vi "SSFG_simple.vi"() -> ()   [LabVIEW 2014]
uses:
  <vilib>/Utility/error.llb/DialogType.ctl
  <vilib>/DAQmx/write.llb/DAQmx Write (Analog Wfm 1Chan NSamp).vi
  <vilib>/DAQmx/create/channels.llb/DAQmx Create Channel (AO-Voltage-Basic).vi
  <vilib>/DAQmx/configure/timing.llb/DAQmx Timing (Sample Clock).vi
  <vilib>/DAQmx/miscellaneous.llb/DAQmx Fill In Error Info.vi
  <resource>/objmgr/daqmx.rc
  <vilib>/measure/NI_MABase.lvlib
panel:
  out "Waveform Graph 2":waveform(dbl)(graph)
  in  "Power Signal Parameters":T1={"Waveform Type"=0, "Amplitude"=1.0, "Frequency"=17.0} {"Frequency" format="%0.2p"; "Waveform Type" items=["Sine Wave", "Triangle Wave", "Square Wave", "Sawtooth Wave"]}
  in  "Number of Samples/Cycle":dbl=1000.0
  in  "Stop":bool
  in  "Update Rate":dbl=1000.0 format="%0.2f"
  in  "Physical Channel":tag
  in  "Power Signal":bool
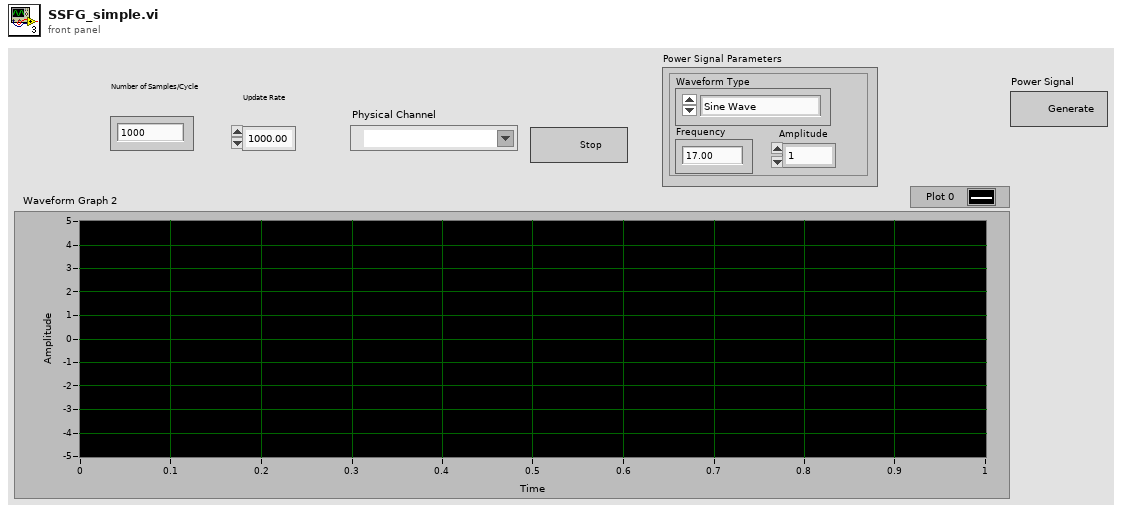
[diagram p1: front panel]
types:
  T1 = cluster{"Waveform Type":u16, "Amplitude":dbl, "Frequency":dbl}
  T2 = typedef "DialogType.ctl" = u16
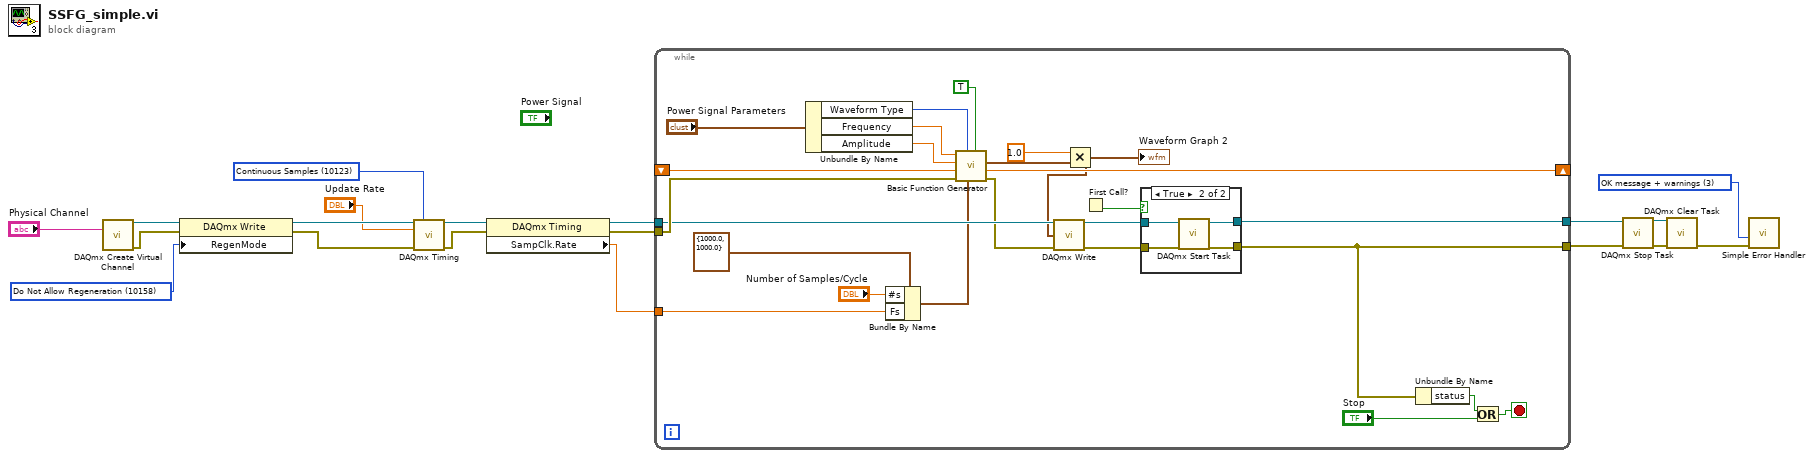
[diagram p0: block diagram]
diagram:
  w8 = T2 3 items=["no dialog", "OK message", "continue or stop message", "OK message + warnings", "continue/stop + warnings"] ("type of dialog (OK msg:1)")
  w13 = 10123 items=["Finite Samples"=10178, "Continuous Samples"=10123, "Hardware Timed Single Point"=12522] ("sample mode")
  w14 = 10158 items=["Allow Regeneration"=10097, "Do Not Allow Regeneration"=10158] ("RegenMode")
  n1 = call-poly <vilib>:"DAQmx Create Virtual Channel.vi"("physical channels"="Physical Channel") -> ("task out"=w18:refnum<k21>, "error out"=w16:errorcluster)  [unwired: 13 in]
  n2 = property class="DAQmx Write"(reference=w18, error in=w16, "RegenMode"=w14) -> (reference out=w17:refnum<k21>, error out=w15:errorcluster)
  n3 = call-poly <vilib>:"DAQmx Timing.vi"("task/channels in"=w17, "sample mode"=w13, "rate"="Update Rate", "error in"=w15) -> ("task out"=w11:refnum<k21>, "error out"=w10:errorcluster)  [unwired: 10 in]
  n4 = property class="DAQmx Timing"(reference=w11, error in=w10) -> (reference out=w2:refnum<k21>, error out=w1:errorcluster, "SampClk.Rate"=w9:dbl)
  n5 = while "while" {
    tunnel: w1 -> [w44]
    tunnel: w9 -> [w42]
    tunnel: w2 -> [w41]
    tunnel: [w36] -> w4
    tunnel: [w35] -> w3
    shift-right: [w23] -> _
    shift-left: _ -> [w22]
    stop <- w33 stop-if-true
    n6 = Unbundle By Name("Power Signal Parameters") -> ("Waveform Type"=w29:u16, "Frequency"=w28:dbl, "Amplitude"=w27:dbl)
    n7 = Bundle By Name(cluster=cluster{"Fs":dbl, "#s":dbl} {"Fs"=1000.0, "#s"=1000.0} ("sampling info"), "#s"="Number of Samples/Cycle", "Fs"=w42) -> (w30:cluster{"Fs":dbl, "#s":dbl})
    n8 = call <vilib>:"Basic Function Generator.vi"("reset signal"=TRUE, "sampling info"=w30, "signal type"=w29, "error in (no error)"=w44, "phase"=w22, "amplitude"=w27, "frequency"=w28) -> ("error out"=w38:errorcluster, "phase out"=w23:dbl, "signal out"=w25:waveform(dbl))  [unwired: 2 in]
    n9 = Multiply(x=1.0 ("y"), y=w25) -> (x*y=w20:waveform(dbl))
    "Waveform Graph 2" <- w20
    n10 = call-poly <vilib>:"DAQmx Write.vi"("task/channels in"=w41, "data"=w20, "error in"=w38) -> ("task out"=w40:refnum<k21>, "error out"=w39:errorcluster)  [unwired: 10 in, 1 out]
    n11 = First Call?() -> (First Call?: T/F=w37:bool)
    n12 = case shown="True" w37 {
      tunnel: w40 -> [w45 w50]
      tunnel: w39 -> [w46 w49]
      tunnel: [w45 w48] -> w36
      tunnel: [w46 w47] -> w35
      frame False {
      }
      frame True {
        n13 = call <vilib>:"DAQmx Start Task.vi"("task/channels in"=w50, "error in"=w49) -> ("task out"=w48:refnum<k21>, "error out"=w47:errorcluster)  [unwired: 12 in]
      }
    }
    n14 = Unbundle By Name(w35) -> ("status"=w32:bool)
    n15 = Or(x=w32, y="Stop") -> (x .or. y?=w33:bool)
  }
  n16 = call <vilib>:"DAQmx Stop Task.vi"("task/channels in"=w4, "error in"=w3) -> ("task out"=w6:refnum<k21>, "error out"=w7:errorcluster)  [unwired: 12 in]
  n17 = call <vilib>:"DAQmx Clear Task.vi"("task in"=w6, "error in"=w7) -> ("error out"=w5:errorcluster)  [unwired: 13 in]
  n18 = call <vilib>:"Simple Error Handler.vi"("type of dialog (OK msg:1)"=w8, "error in (no error)"=w5) -> ()  [unwired: 3 in, 5 out]
